vi "saveLogEntry.vi"(8 "error in (no error)":errorcluster, 11 "Logger in":refnum<class "TestDataLog.lvclass">) -> (0 "error out":errorcluster, 3 "Logger out":refnum<class "TestDataLog.lvclass">)   [LabVIEW 2013, in "TestDataLog.lvclass"]
uses:
  TestDataLog.lvclass
  TestDataLog.lvclass/TestDataLog.ctl
  Log/Log.lvclass/Log.ctl
  Log/Log.lvclass
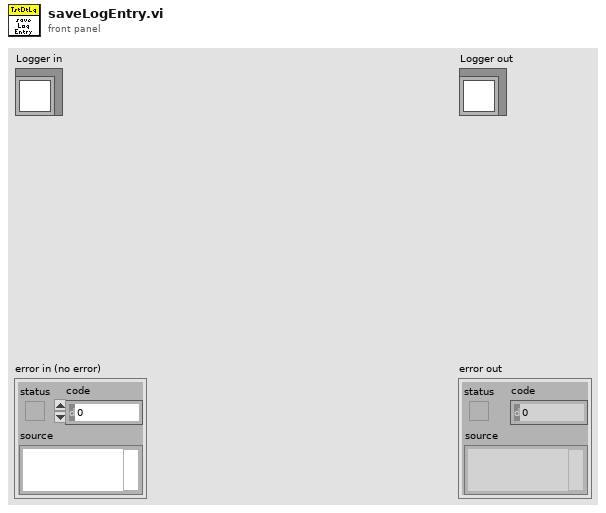
[diagram p1: front panel]
types:
  T1 = typedef "M2AADTTypedefs.lvlib/InputData.ctl" = cluster{"Limit Switches":T2, "SSI Encoder":i32, "Force Measured":T3, "Distance Data":T4, "Thermocouple Data":T5}
  T2 = typedef "ILCCommon.lvlib/ILCTypedefs.lvlib/LimitSwitches.ctl" = cluster{"1":bool, "2":bool}
  T3 = typedef "M2AADTTypedefs.lvlib/ForceDemand.ctl" = dbl[unit]
  T4 = typedef "M2AADTTypedefs.lvlib/Distance Data.ctl" = cluster{"Distance Measured 1":dbl[unit], "Distance Measured 2":dbl[unit]}
  T5 = typedef "M2AADTTypedefs.lvlib/ThermocoupleData.ctl" = cluster{"Motor Temperature":dbl[unit]}
  T6 = typedef "M2AADTTypedefs.lvlib/ControllerData.ctl" = cluster{"Force Demand":T3, "Force Error":T3}
  T7 = typedef "M2AADTTypedefs.lvlib/OutputData.ctl" = cluster{"Step & Direction":i16}
  T8 = typedef "M2AADTTypedefs.lvlib/StateSelector.ctl" = enum16{"EndingCycleState", "FaultState", "InteractiveMotionState", "MovingToNewForceState", "OffState", "PausingState", "StandbyState", "StoppedState"}
  T9 = typedef "M2AADTTypedefs.lvlib/TestStatus.ctl" = cluster{"activeCycle":u32, "activeProfileStep":u32}
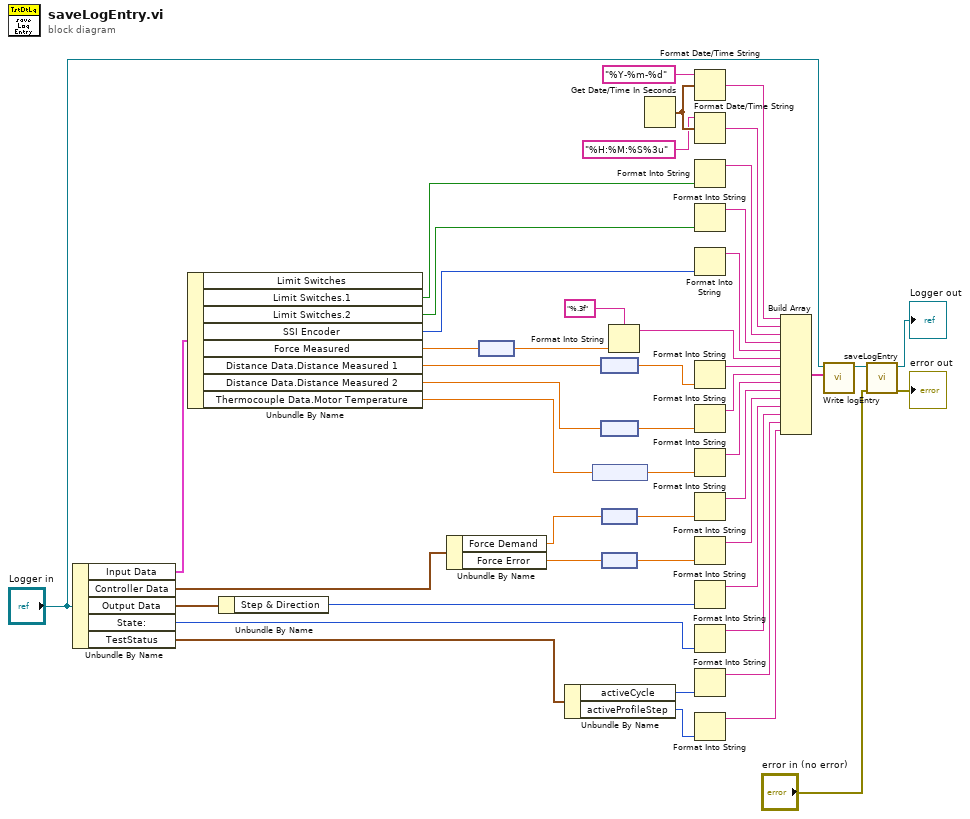
[diagram p0: block diagram]
diagram:
  n1 = Unbundle By Name("Logger in") -> ("Input Data"=w48:T1, "Controller Data"=w47:T6, "Output Data"=w34:T7, "State:"=w31:T8, "TestStatus"=w16:T9)
  n2 = Unbundle By Name(w48) -> ("Limit Switches.1"=w46:bool, "Limit Switches.2"=w44:bool, "SSI Encoder"=w42:i32, "Force Measured"=w28:T3, "Distance Data.Distance Measured 1"=w26:dbl[unit], "Distance Data.Distance Measured 2"=w24:dbl[unit], "Thermocouple Data.Motor Temperature"=w22:dbl[unit])  [unwired: 1 out]
  n3 = Unbundle By Name(w34) -> ("Step & Direction"=w33:i16)
  n4 = Unbundle By Name(w47) -> ("Force Demand"=w20:T3, "Force Error"=w18:T3)
  n5 = node(w28) -> (w27:dbl)
  n6 = Unbundle By Name(w16) -> ("activeCycle"=w15:u32, "activeProfileStep"=w14:u32)
  n7 = node(w22) -> (w21:dbl)
  n8 = node(w26) -> (w25:dbl)
  n9 = node(w24) -> (w23:dbl)
  n10 = node(w20) -> (w19:dbl)
  n11 = node(w18) -> (w17:dbl)
  n12 = Format Into String(format string="%.3f", w27) -> (resulting string=w40:string)  [unwired: 2 in, 1 out]
  n13 = Get Date/Time In Seconds() -> (seconds since 1Jan1904=w10:timestamp)
  n14 = Format Date/Time String(time format string (%c)="%Y-%m-%d" ("format string"), seconds (now)=w10) -> (date/time string=w7:string)  [unwired: 1 in]
  n15 = Format Date/Time String(time format string (%c)="%H:%M:%S%3u", seconds (now)=w10) -> (date/time string=w8:string)  [unwired: 1 in]
  n16 = Format Into String(w46) -> (resulting string=w45:string)  [unwired: 3 in, 1 out]
  n17 = Format Into String(w44) -> (resulting string=w43:string)  [unwired: 3 in, 1 out]
  n18 = Format Into String(w42) -> (resulting string=w41:string)  [unwired: 3 in, 1 out]
  n19 = Format Into String(w25) -> (resulting string=w39:string)  [unwired: 3 in, 1 out]
  n20 = Format Into String(w23) -> (resulting string=w38:string)  [unwired: 3 in, 1 out]
  n21 = Format Into String(w21) -> (resulting string=w37:string)  [unwired: 3 in, 1 out]
  n22 = Format Into String(w19) -> (resulting string=w36:string)  [unwired: 3 in, 1 out]
  n23 = Format Into String(w17) -> (resulting string=w35:string)  [unwired: 3 in, 1 out]
  n24 = Format Into String(w33) -> (resulting string=w32:string)  [unwired: 3 in, 1 out]
  n25 = Format Into String(w31) -> (resulting string=w30:string)  [unwired: 3 in, 1 out]
  n26 = Format Into String(w15) -> (resulting string=w13:string)  [unwired: 3 in, 1 out]
  n27 = Format Into String(w14) -> (resulting string=w12:string)  [unwired: 3 in, 1 out]
  n28 = Build Array(w7, w8, w45, w43, w41, w40, w39, w38, w37, w36, w35, w32, w30, w13, w12) -> (w4:string[])
  n29 = call "Write logEntry.vi"("logEntry"=w4, "Logger in"="Logger in") -> ("Logger out"=w5:refnum<class "TestDataLog.lvclass">)  [unwired: 9 in]
  n30 = call-parent "saveLogEntry.vi"("error in (no error)"="error in (no error)", "Logger in"=w5) -> ("error out"=→"error out":errorcluster, "Logger out"=→"Logger out":refnum<class "TestDataLog.lvclass">)  [unwired: 8 in]
